vi "Subtract Background Image (SubVI).vi"(0 "Pixels In":u64, 1 "BG SUB TH":i16, 2 "Subtract BG":bool, 3 "Mode":bool, 11 "Input Valid":bool) -> (4 "Pixels Out":u64, 15 "Output Valid":bool)   [LabVIEW 2015]
uses:
  <vilib>/rvi/DataTransferAndStorage/Container/XNode/niFpgaContainer.xnode
  <vilib>/rvi/FIFO/Fifo_Resource/nirvififoEmulationRead.vi
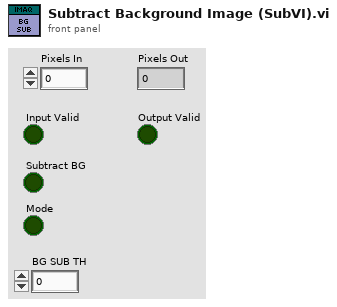
[diagram p1: front panel]
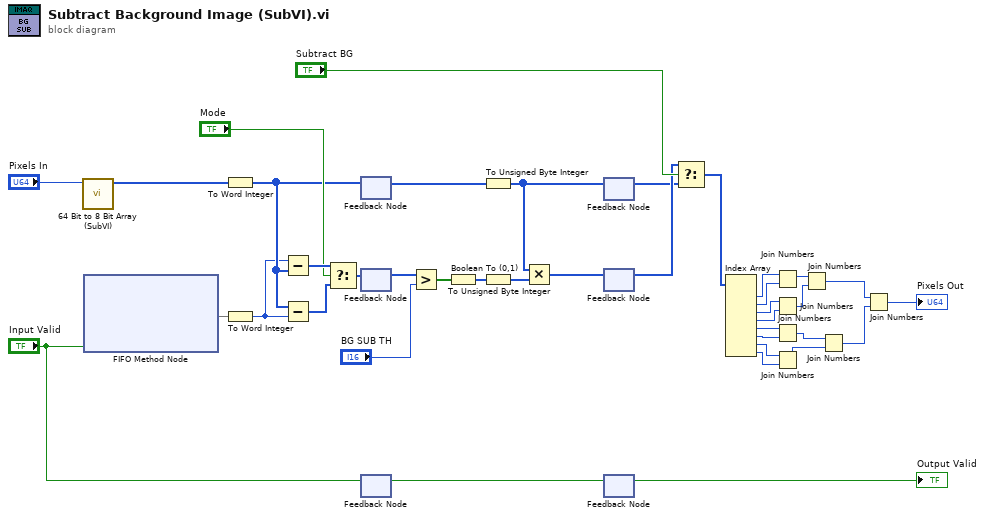
[diagram p0: block diagram]
diagram:
  n1 = call "64 Bit to 8 Bit Array (SubVI).vi"("Pixel In"="Pixels In") -> ("Pixel Array Out"=w8:u8[])  [unwired: 10 in]
  n2 = xnode ("FIFO Method Node")("Ready for Output"="Input Valid") -> ("Element"=w17)  [unwired: 1 in, 2 out]
  n3 = To Word Integer(number=w8) -> (16bit integer=w4:i16[])
  n4 = To Word Integer(number=w17) -> (16bit integer=w3:i16)
  n5 = Subtract(x=w3, y=w4) -> (x-y=w16:i16[])
  n6 = Subtract(x=w4, y=w3) -> (x-y=w15:i16[])
  n7 = Select(t=w16, s="Mode", f=w15) -> (s? t:f=w14:i16[])
  n8 = feedback-in #1(w4) -> ()
  n9 = feedback #1() -> (w7:i16[])  [unwired: 1 in]
  n10 = feedback-in #2(w14) -> ()
  n11 = feedback #2() -> (w6:i16[])  [unwired: 1 in]
  n12 = feedback-in #3("Input Valid") -> ()
  n13 = feedback #3() -> (w5:bool)  [unwired: 1 in]
  n14 = Greater?(x=w6, y="BG SUB TH") -> (0:w12:bool[])
  n15 = Boolean To (0,1)(Boolean=w12) -> (0, 1=w11:i16[])
  n16 = To Unsigned Byte Integer(number=w7) -> (unsigned 8bit integer=w2:u8[])
  n17 = To Unsigned Byte Integer(number=w11) -> (unsigned 8bit integer=w10:u8[])
  n18 = Multiply(x=w2, y=w10) -> (x*y=w9:u8[])
  n19 = feedback-in #4(w2) -> ()
  n20 = feedback #4() -> (w20:u8[])  [unwired: 1 in]
  n21 = feedback-in #5(w9) -> ()
  n22 = feedback #5() -> (w21:u8[])  [unwired: 1 in]
  n23 = feedback #6() -> (→"Output Valid":bool)  [unwired: 1 in]
  n24 = feedback-in #6(w5) -> ()
  n25 = Select(t=w21, s="Subtract BG", f=w20) -> (s? t:f=w38:u8[])
  n26 = Index Array(array=w38) -> (element #1=w23:u8, element #2=w24:u8, element #3=w25:u8, element #4=w26:u8, element #5=w27:u8, element #6=w28:u8, element #7=w29:u8, element #8=w30:u8)  [unwired: 8 in]
  n27 = Join Numbers(hi=w23, lo=w24) -> ((hi.lo)=w33:u16)
  n28 = Join Numbers(hi=w25, lo=w26) -> ((hi.lo)=w34:u16)
  n29 = Join Numbers(hi=w27, lo=w28) -> ((hi.lo)=w31:u16)
  n30 = Join Numbers(hi=w29, lo=w30) -> ((hi.lo)=w32:u16)
  n31 = Join Numbers(hi=w33, lo=w34) -> ((hi.lo)=w35:u32)
  n32 = Join Numbers(hi=w31, lo=w32) -> ((hi.lo)=w36:u32)
  n33 = Join Numbers(hi=w35, lo=w36) -> ((hi.lo)=→"Pixels Out":u64)
